vi "Loader.vi"(9 "Loader Name":string, 10 "PID":u32) -> ()   [LabVIEW 2021, in "CIFPluginLoader.lvclass"]
uses:
  CIFPluginLoader.lvclass
  <vilib>/CIF Foundation/CIF Core/CIFUtilities/CIFLogs/Typedef/Message Type.ctl
  gRPC/CIF_PluginLoader_server/RPC Messages/cif_pluginloader_DiscoverResponse.ctl
  gRPC/CIF_PluginLoader_server/RPC Messages/cif_pluginloader_DiscoveredPlugin.ctl
  gRPC/CIF_PluginLoader_server/RPC Messages/cif_common_Version.ctl
  gRPC/CIF_PluginLoader_server/RPC Messages/cif_management_common_PluginMetadata.ctl
  gRPC/CIF_PluginLoader_server/RPC Messages/cif_common_Status.ctl
  CIFPluginLoader.lvclass/CIFPluginLoader.ctl
  gRPC/CIF_PluginLoader_server/RPC Messages/cif_pluginloader_DestroyResponse.ctl
  <vilib>/CIF Foundation/CIF Core/CIFCore/Common/Typedef/Errors.ctl
  gRPC/CIF_PluginLoader_server/RPC Messages/cif_pluginloader_LoadPluginResponse.ctl
  gRPC/CIF_PluginLoader_server/RPC Messages/cif_pluginloader_AbortPluginResponse.ctl
  gRPC/CIF_PluginLoader_server/RPC Messages/cif_pluginloader_PingResponse.ctl
  gRPC/CIF_PluginLoader_server/RPC Messages/cif_management_common_LoaderInfoFull.ctl
  gRPC/CIF_PluginLoader_server/RPC Messages/cif_management_common_LoaderType.ctl
  9a3a4a83-316c-4994-a2ad-738e23b33a77.vi
  903a1d06-a2f6-408e-a72e-d05a96790f6b.vi
  gRPC/CIF_PluginLoader_server/RPC Messages/Get cif_pluginloader_DestroyRequest.vi
  gRPC/CIF_PluginLoader_server/RPC Messages/Set cif_pluginloader_DestroyResponse.vi
  gRPC/CIF_PluginLoader_server/RPC Messages/Get cif_pluginloader_LoadPluginRequest.vi
  gRPC/CIF_PluginLoader_server/RPC Messages/Set cif_pluginloader_LoadPluginResponse.vi
  <vilib>/CIF Foundation/CIF Utilities/Errors/Append Error Location.vi
  gRPC/CIF_PluginLoader_server/RPC Messages/Get cif_pluginloader_AbortPluginRequest.vi
  gRPC/CIF_PluginLoader_server/RPC Messages/Set cif_pluginloader_AbortPluginResponse.vi
  gRPC/CIF_PluginLoader_server/RPC Messages/Get cif_pluginloader_PingRequest.vi
  gRPC/CIF_PluginLoader_server/RPC Messages/Set cif_pluginloader_PingResponse.vi
  gRPC/CIF_PluginLoader_server/RPC Messages/Get cif_pluginloader_DiscoverRequest.vi
  gRPC/CIF_PluginLoader_server/RPC Messages/Set cif_pluginloader_DiscoverResponse.vi
  <vilib>/Utility/High Resolution Relative Seconds.vi
  gRPC/CIF_PluginLoader_server/RPC Messages/Get cif_pluginloader_DestroyRequest.vi/2ed25e12-861d-4677-8ead-ace2906b2041.vi
  gRPC/CIF_PluginLoader_server/RPC Messages/FlatToRichcif_pluginloader_DestroyRequest.vi
  gRPC/CIF_PluginLoader_server/RPC Messages/Set cif_pluginloader_DestroyResponse.vi/dcc74a39-081a-4bdd-860b-8ed792803c96.vi
  gRPC/CIF_PluginLoader_server/RPC Messages/RichToFlatcif_pluginloader_DestroyResponse.vi
  gRPC/CIF_PluginLoader_server/RPC Messages/Get cif_pluginloader_LoadPluginRequest.vi/2ed25e12-861d-4677-8ead-ace2906b2041.vi
  gRPC/CIF_PluginLoader_server/RPC Messages/FlatToRichcif_pluginloader_LoadPluginRequest.vi
  gRPC/CIF_PluginLoader_server/RPC Messages/Set cif_pluginloader_LoadPluginResponse.vi/dcc74a39-081a-4bdd-860b-8ed792803c96.vi
  gRPC/CIF_PluginLoader_server/RPC Messages/RichToFlatcif_pluginloader_LoadPluginResponse.vi
  gRPC/CIF_PluginLoader_server/RPC Messages/Get cif_pluginloader_AbortPluginRequest.vi/2ed25e12-861d-4677-8ead-ace2906b2041.vi
  gRPC/CIF_PluginLoader_server/RPC Messages/FlatToRichcif_pluginloader_AbortPluginRequest.vi
  gRPC/CIF_PluginLoader_server/RPC Messages/Set cif_pluginloader_AbortPluginResponse.vi/dcc74a39-081a-4bdd-860b-8ed792803c96.vi
  gRPC/CIF_PluginLoader_server/RPC Messages/RichToFlatcif_pluginloader_AbortPluginResponse.vi
  gRPC/CIF_PluginLoader_server/RPC Messages/Get cif_pluginloader_PingRequest.vi/2ed25e12-861d-4677-8ead-ace2906b2041.vi
  gRPC/CIF_PluginLoader_server/RPC Messages/FlatToRichcif_pluginloader_PingRequest.vi
  gRPC/CIF_PluginLoader_server/RPC Messages/Set cif_pluginloader_PingResponse.vi/dcc74a39-081a-4bdd-860b-8ed792803c96.vi
  gRPC/CIF_PluginLoader_server/RPC Messages/RichToFlatcif_pluginloader_PingResponse.vi
  gRPC/CIF_PluginLoader_server/RPC Messages/Get cif_pluginloader_DiscoverRequest.vi/2ed25e12-861d-4677-8ead-ace2906b2041.vi
  gRPC/CIF_PluginLoader_server/RPC Messages/FlatToRichcif_pluginloader_DiscoverRequest.vi
  gRPC/CIF_PluginLoader_server/RPC Messages/Set cif_pluginloader_DiscoverResponse.vi/dcc74a39-081a-4bdd-860b-8ed792803c96.vi
  gRPC/CIF_PluginLoader_server/RPC Messages/RichToFlatcif_pluginloader_DiscoverResponse.vi
  <vilib>/gRPC/LabVIEW gRPC Library/Shared/TranslateGrpcError.vi
  gRPC/CIF_PluginLoader_server/RPC Messages/RichToFlatcif_common_Status.vi
  gRPC/CIF_PluginLoader_server/RPC Messages/RichToFlatcif_management_common_LoaderInfoFull.vi
  gRPC/CIF_PluginLoader_server/RPC Messages/RichToFlatcif_pluginloader_DiscoveredPlugin.vi
  gRPC/CIF_PluginLoader_server/RPC Messages/RichToFlatcif_common_Version.vi
  gRPC/CIF_PluginLoader_server/RPC Messages/RichToFlatcif_management_common_PluginMetadata.vi
  <vilib>/gRPC/LabVIEW gRPC Library/Server API/Server/Get Server DLL Path.vi
  <vilib>/Utility/error.llb/Error Cluster From Error Code.vi
  <vilib>/gRPC/LabVIEW gRPC Library/Server API/Message Requests/Complete Call.vi
  <vilib>/gRPC/LabVIEW gRPC Servicer/Servicer/Servicer.lvclass
  <vilib>/CIF Foundation/CIF Core/CIFUtilities/CIFLogs/CIFLogs.lvlib
  <vilib>/Utility/LVLibp/NI_PackedLibraryUtility.lvlib
  gRPC/CIF_PluginLoader_server/RPC Service/PluginLoader/PluginLoader.lvclass
  gRPC/CIF_PluginLoader_server/CIF_PluginLoader_server.lvlib
  gRPC/CIF_Plugin_Loader_Client_Wrapper/CIFPluginLoaderClientWrapper.lvlib
  <vilib>/CIF Foundation/CIF Core/CIFCore/Common/CIFCoreCommon.lvlib
panel:
  out "error out":errorcluster
  in  "stop":bool
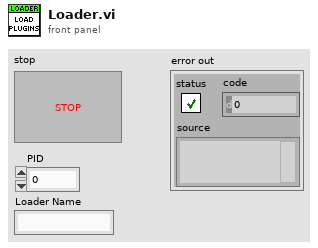
[diagram p1: front panel]
types:
  T1 = typedef "CIFLogs.lvlib/Message Type.ctl" = enum16{"Error", "Information", "Print Terminal", "Configuration"}
  T2 = typedef "CIF_PluginLoader_server.lvlib/cif_pluginloader_DiscoverResponse.ctl" = cluster{"discovered_plugins":T3[], "status":T6}
  T3 = typedef "CIF_PluginLoader_server.lvlib/cif_pluginloader_DiscoveredPlugin.ctl" = cluster{"file_path":string, "file_name":string, "plugin_type":string, "plugin_version":T4, "plugin_metadata":T5, "relative_path":string[]}
  T4 = typedef "CIF_PluginLoader_server.lvlib/cif_common_Version.ctl" = cluster{"major":u32, "minor":u32, "fix":u32, "build":u32}
  T5 = typedef "CIF_PluginLoader_server.lvlib/cif_management_common_PluginMetadata.ctl" = cluster{"description":string, "history":string, "author":string}
  T6 = typedef "CIF_PluginLoader_server.lvlib/cif_common_Status.ctl" = cluster{"code":i32, "message":string}
  T7 = typedef "CIF_PluginLoader_server.lvlib/cif_pluginloader_DestroyResponse.ctl" = cluster{"void":string}
  T8 = typedef "CIFCoreCommon.lvlib/Errors.ctl" = enum16{"Invalid Clock ID", "Long Sleep", "gRPC Server Not Found", "Config Parse", "Timestamp Wrap", "Delayed Execution", "Duplicate Channel", "Missing Channel", "Incorrect Type", "Flatten Error", "Unflatten Data", "Unique Name", "Plugin Not Found", "Plugin Type Not Found", "Plugin Version Not Found", "Manager Not Found", "Numerical Issue", "Time Jump", "Clock ID Match", "Channel Length", "Plugin Connection", "gRPC Server Connection", "PPL Name Match", "Build", "Config Log Parse", "Plugin Load", "UI Subpanel Load", "Python Name", "Invalid Name", "Unable to Change Ch Buffer", "Failed Kill", "Failed SysExec", "Function Not Implemented", "Load Timeout"}
  T9 = typedef "CIF_PluginLoader_server.lvlib/cif_pluginloader_LoadPluginResponse.ctl" = cluster{"status":T6}
  T10 = typedef "CIF_PluginLoader_server.lvlib/cif_pluginloader_AbortPluginResponse.ctl" = cluster{"status":T6}
  T11 = typedef "CIF_PluginLoader_server.lvlib/cif_pluginloader_PingResponse.ctl" = cluster{"loader_info":T12}
  T12 = typedef "CIF_PluginLoader_server.lvlib/cif_management_common_LoaderInfoFull.ctl" = cluster{"loader_type":T13, "loader_name":string, "grpc_port":i32, "pid":u32}
  T13 = typedef "CIF_PluginLoader_server.lvlib/cif_management_common_LoaderType.ctl" = enum32{"LOADERTYPE_UNKNOWN", "LOADERTYPE_LABVIEW"}
  T14 = typedef "grpc-lvsupport-release.lvlib/grpcId.ctl" = u64
  T15 = typedef "CIF_PluginLoader_server.lvlib/cif_pluginloader_LoadPluginRequest.ctl" = cluster{"plugin_name":string, "path":string}
  T16 = typedef "CIFPluginLoader.lvclass/Loaded Plugin Map.ctl" = map{string, refnum<vi>}
  T17 = typedef "CIF_PluginLoader_server.lvlib/cif_pluginloader_AbortPluginRequest.ctl" = cluster{"plugin_name":string}
  T18 = typedef "CIF_Manager_client.lvlib/cif_management_common_LoaderType.ctl" = enum32{"LOADERTYPE_UNKNOWN", "LOADERTYPE_LABVIEW"}
  T19 = typedef "CIF_PluginLoader_server.lvlib/cif_pluginloader_DiscoverRequest.ctl" = cluster{"update_metadata":bool}
  T20 = typedef "CIFPluginManager.lvclass/Discovered Plugin.ctl" = cluster{"Filename":string, "Plugin Type":string, "Qualified name":string, "Version":T21, "Plugin Metadata":T22, "Loader Type":T23, "File Path":string, "Relative Path":string[]}
  T21 = typedef "CIFCoreCommon.lvlib/Version.ctl" = cluster{"Major":i32, "Minor":i32, "Fix":i32, "Build":i32}
  T22 = typedef "CIFPluginManager.lvclass/Plugin Metadata.ctl" = cluster{"Description":string, "History":string, "Author":string}
  T23 = typedef "CIFPluginManager.lvclass/Loader Type.ctl" = enum16{"LabVIEW"}
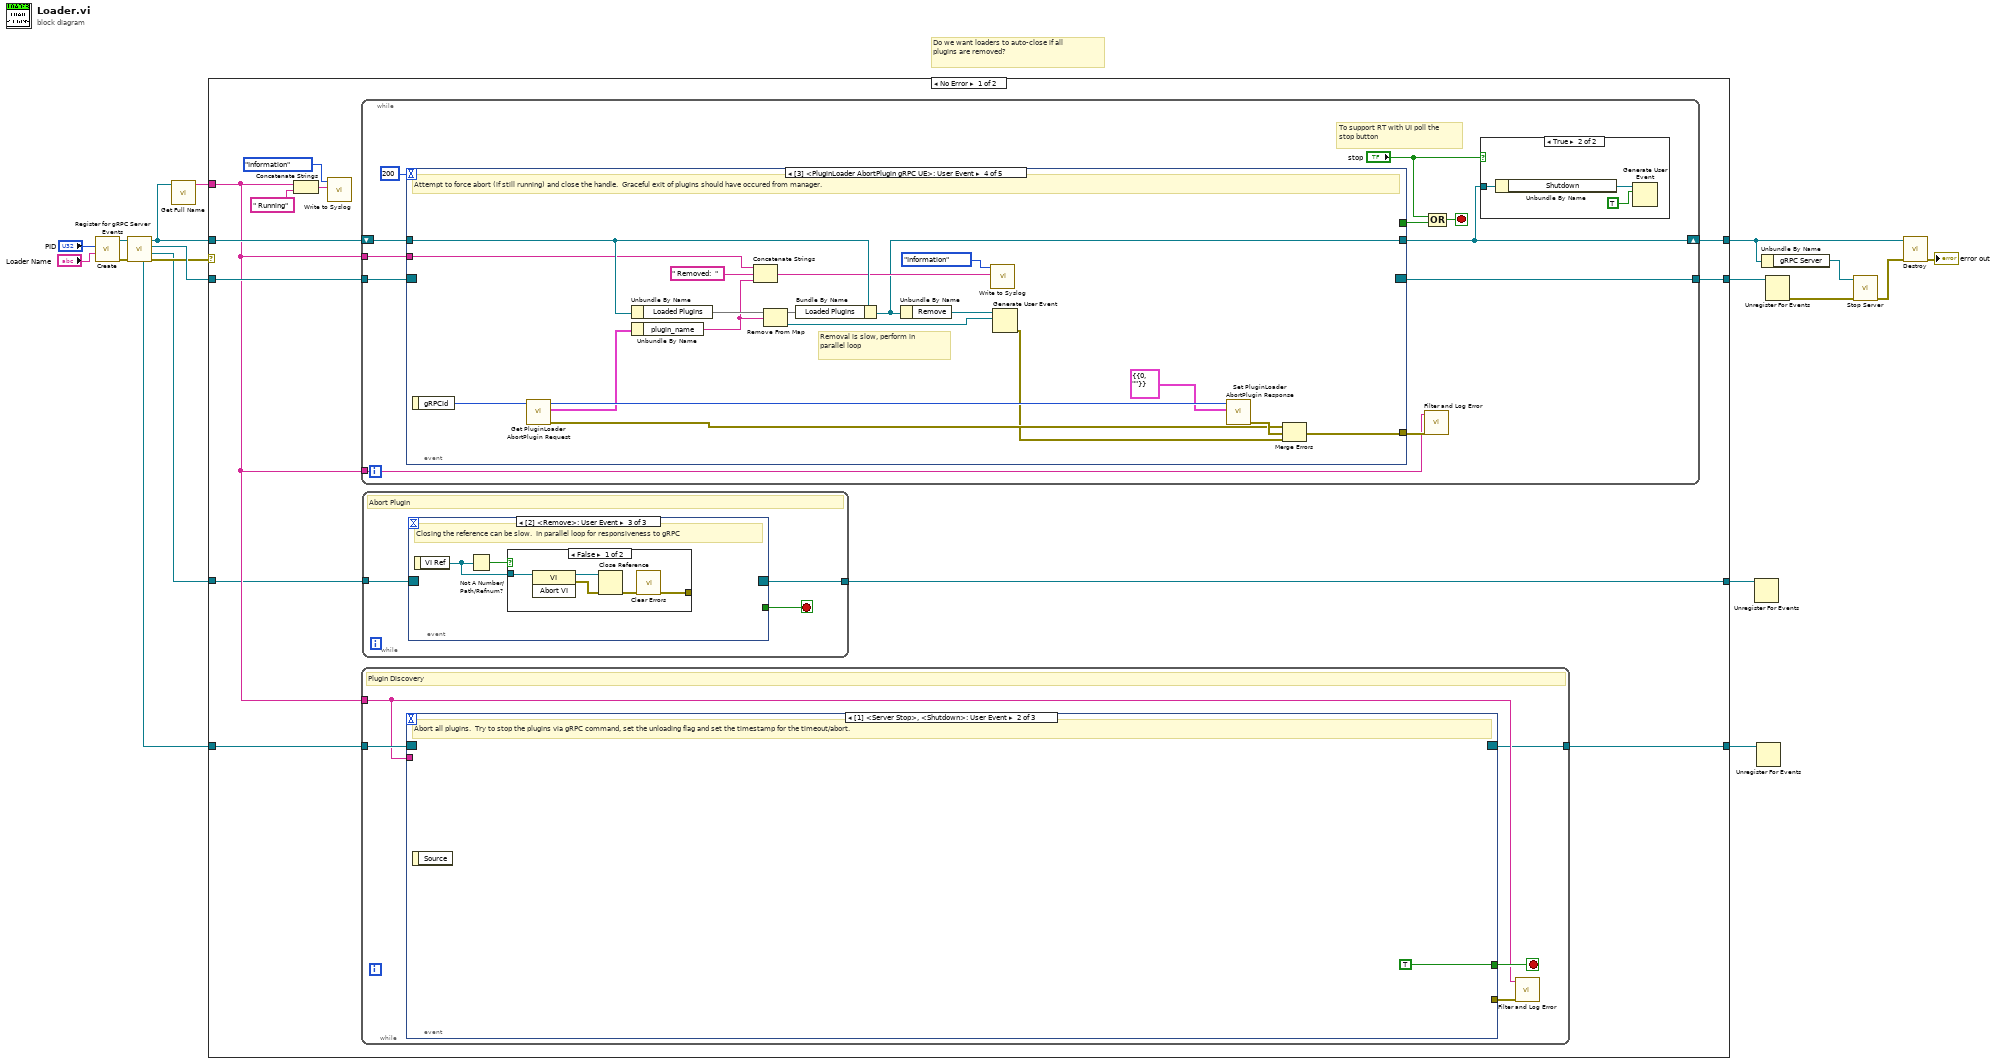
[diagram p0: block diagram]
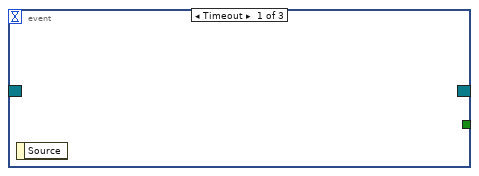
[diagram p2: hidden frame]
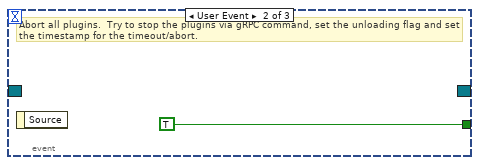
[diagram p3: hidden frame]
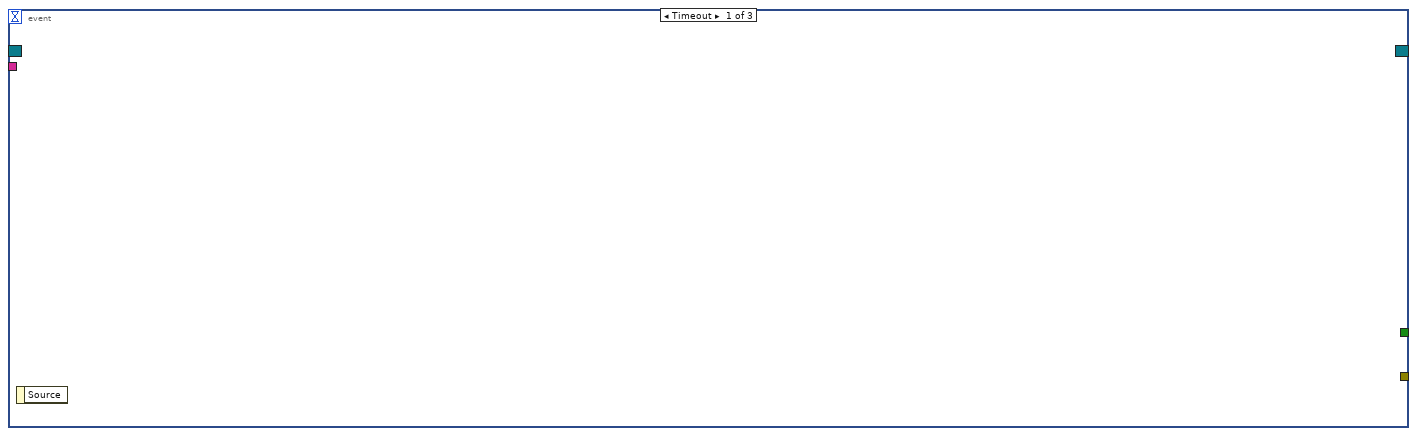
[diagram p5: hidden frame]
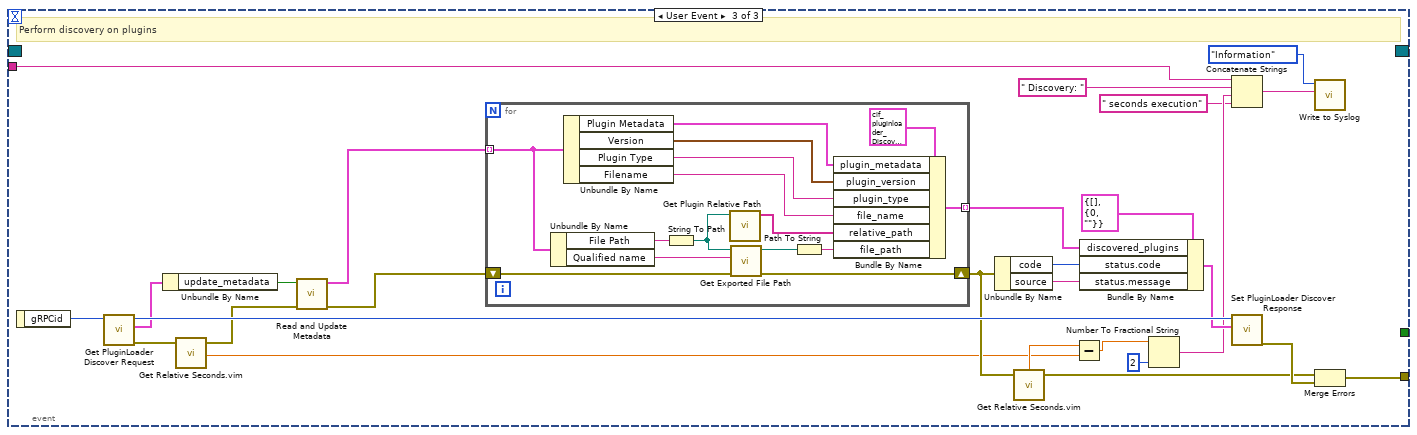
[diagram p6: hidden frame]
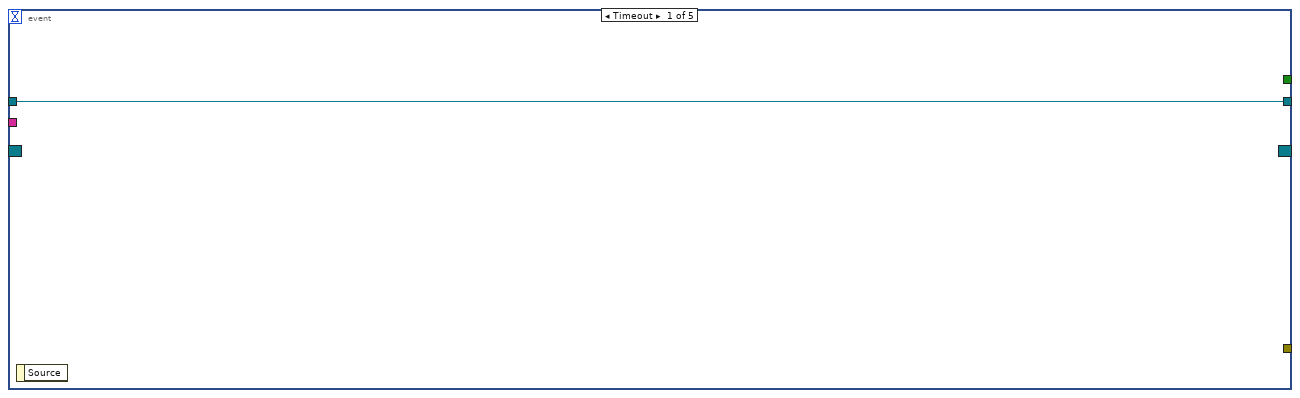
[diagram p8: hidden frame]
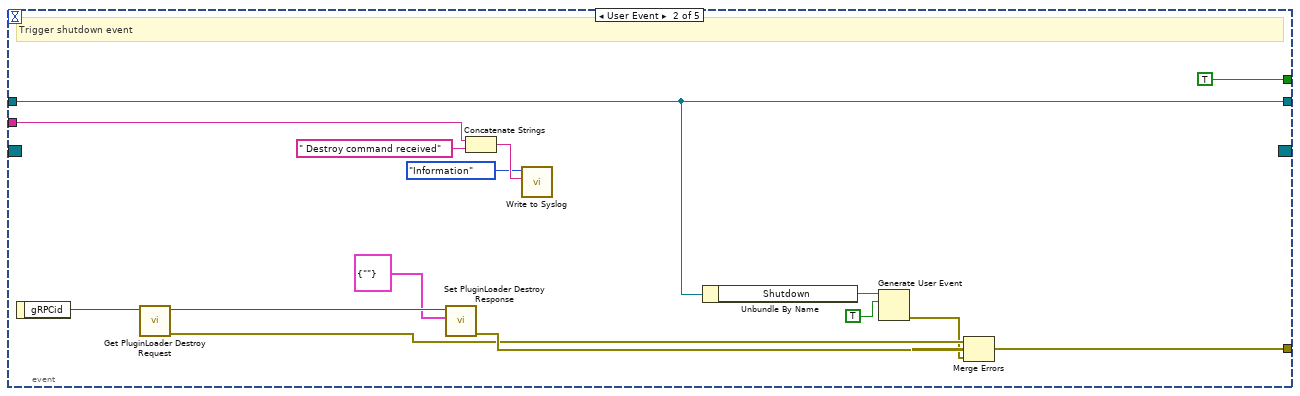
[diagram p9: hidden frame]
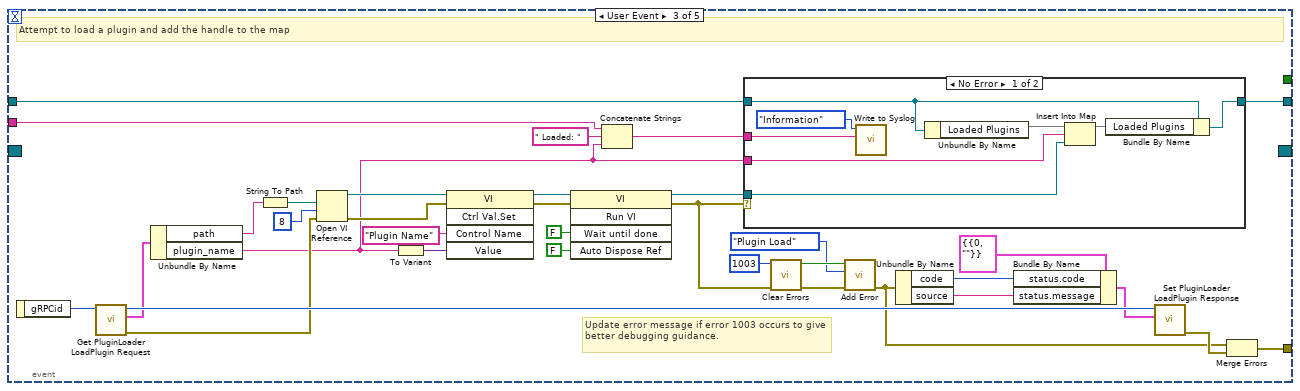
[diagram p10: hidden frame]
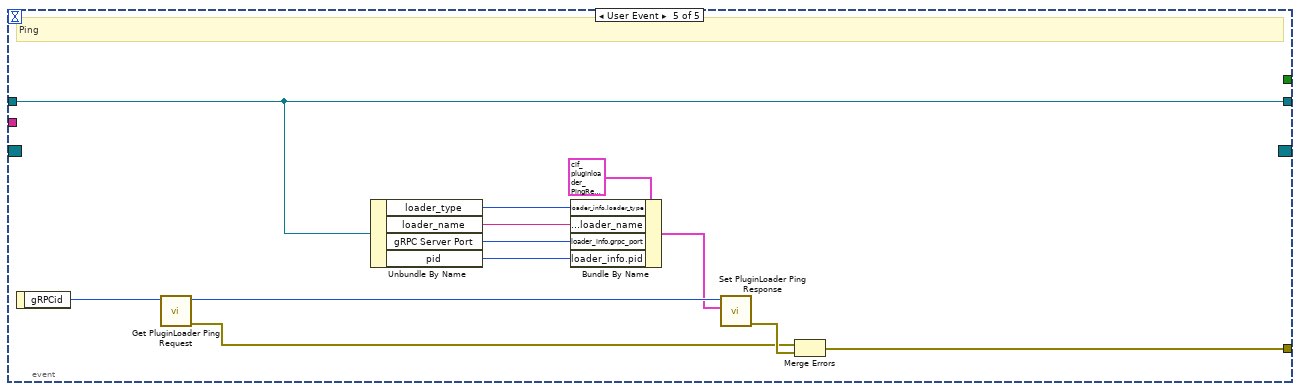
[diagram p12: hidden frame]
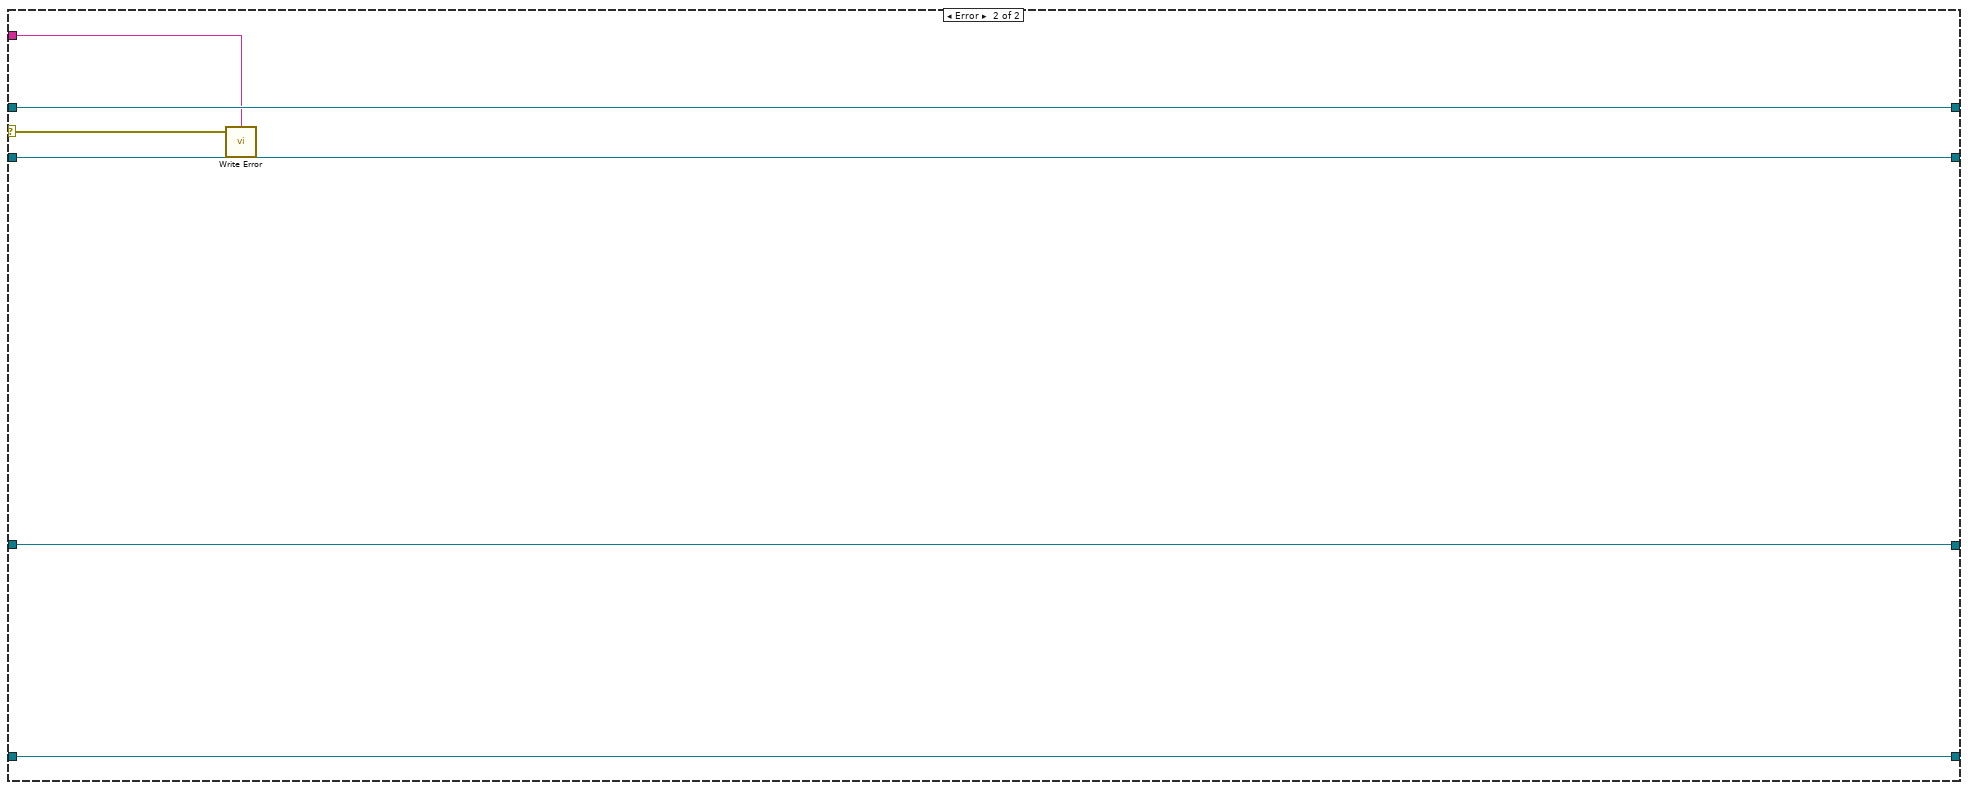
[diagram p13: hidden frame]
diagram:
  # "Do we want loaders to auto-close if all plugins are removed?"
  n1 = call "Create.vi"("Loader Name"="Loader Name", "pid"="PID") -> ("error out"=w13:errorcluster, "Plugin Manager out"=w9:refnum<class "CIFPluginLoader.lvclass">)  [unwired: 8 in]
  n2 = call "Register for gRPC Server Events.vi"("error in (no error)"=w13, "CIFLauncher in"=w9) -> ("error out"=w5:errorcluster, "Abort VI Event Registration Refnum"=w3:refnum<event-registration>, "Main Event Registration Refnum"=w12:refnum<event-registration>, "CIFLauncher out"=w7:refnum<class "CIFPluginLoader.lvclass">, "Discovery Event Registration Refnum"=w4:refnum<event-registration>)  [unwired: 5 in]
  n3 = call "Get Full Name.vi"("CIFPluginLoader in"=w7) -> ("Name"=w6:string)  [unwired: 10 in]
  n4 = case shown="No Error" w5 {
    selector: w5 -> [_ w199]
    tunnel: [w30 w198] -> w8
    tunnel: [w29 w197] -> w14
    tunnel: w12 -> [w28 w197]
    tunnel: w7 -> [w27 w198]
    tunnel: w4 -> [w23 w194]
    tunnel: w6 -> [w22 w196]
    tunnel: w3 -> [w19 w195]
    tunnel: [w21 w194] -> w2
    tunnel: [w20 w195] -> w1
    frame No Error {
      n5 = Concatenate Strings(w22, " Running" ("message")) -> (w26:string)
      n6 = call <vilib>:"Write to Syslog.vi"("message"=w26, "CIF Message Type"=Message_Type."Information") -> ()  [unwired: 9 in, 1 out]
      n7 = while {
        tunnel: w28 -> [w95]
        tunnel: [w99] -> w29
        shift-right: [w98] -> w30
        shift-left: w27 -> [w100]
        tunnel: w22 -> [w94]
        tunnel: w22 -> [w93]
        stop <- w91 stop-if-true
        # "To support RT with UI poll the stop button"
        n8 = event shown="[3] <PluginLoader AbortPlugin gRPC UE>: User Event" {
          selector: w95 -> [_ _ _ _ _]
          dyn-events: [_ _ _ _ _] -> w99
          timeout: 200 -> [_ _ _ _ _]
          tunnel: w100 -> [w104 w106 w136 w175 w186]
          tunnel: [w104 w106 w134 w166 w186] -> w98
          tunnel: [_ w119 w138 w177 w190] -> w97
          tunnel: [_ TRUE _ _ _] -> w92
          tunnel: w93 -> [_ w110 w131 w167 _]
          event Timeout {
            n9 = event-data() -> ()  [unwired: 1 in, 1 out]
          }
          event User Event {
            # "Trigger shutdown event"
            n10 = event-data() -> ("gRPCid"=w117:T14)  [unwired: 1 in]
            n11 = call "Get PluginLoader Destroy Request.vi"("gRPCid"=w117) -> ("error out"=w114:errorcluster, "gRPCid out"=w116:T14)  [unwired: 8 in, 1 out]
            n12 = call "Set PluginLoader Destroy Response.vi"("Message Data"=T7 {"void"=""}, "gRPCid in"=w116) -> ("error out"=w115:errorcluster)  [unwired: 9 in]
            n13 = Concatenate Strings(w110, " Destroy command received" ("message")) -> (w113:string)
            n14 = call <vilib>:"Write to Syslog.vi"("message"=w113, "CIF Message Type"=Message_Type."Information") -> ()  [unwired: 9 in, 1 out]
            n15 = Unbundle By Name(w106) -> ("Shutdown"=w108:refnum<user-event>)
            n16 = Generate User Event(user event=w108, event data cluster=TRUE ("event data")) -> (error out=w105:errorcluster)  [unwired: 2 in, 1 out]
            n17 = Merge Errors(w114, w115, w105) -> (w119:errorcluster)
          }
          event User Event {
            # "Update error message if error 1003 occurs to give better debugging guidance."
            # "Attempt to load a plugin and add the handle to the map"
            n18 = event-data() -> ("gRPCid"=w153:T14)  [unwired: 1 in]
            n19 = call "Get PluginLoader LoadPlugin Request.vi"("gRPCid"=w153) -> ("error out"=w140:errorcluster, "Message Data"=w151:T15, "gRPCid out"=w152:T14)  [unwired: 8 in]
            n20 = Unbundle By Name(w151) -> ("path"=w142:string, "plugin_name"=w128:string)
            n21 = String To Path(string=w142) -> (path=w141:path)
            n22 = Open VI Reference(vi path=w141, options=8, error in (no error)=w140) -> (vi reference=w145:refnum<vi>, error out=w148:errorcluster)  [unwired: 3 in]
            n23 = To Variant(anything=w128) -> (Variant=w143:variant)
            n24 = invoke class="VI" method="Ctrl Val.Set"(reference=w145, error in=w148, "Control Name"="Plugin Name", "Value"=w143) -> (reference out=w147:refnum<vi>, error out=w146:errorcluster)  [unwired: 1 in, 3 out]
            n25 = invoke class="VI" method="Run VI"(reference=w147, error in=w146, "Wait until done"=FALSE ("Wait Until Done"), "Auto Dispose Ref"=FALSE ("Auto Dispose Reference")) -> (reference out=w135:refnum<vi>, error out=w121:errorcluster)  [unwired: 1 in, 3 out]
            n26 = Concatenate Strings(w131, " Loaded: " ("message"), w128) -> (w129:string)
            n27 = case shown="No Error" w121 {
              tunnel: w136 -> [w161 w162]
              tunnel: w128 -> [w159 _]
              tunnel: w135 -> [w158 _]
              tunnel: [w156 w162] -> w134
              tunnel: w129 -> [w154 _]
              frame No Error {
                n28 = call <vilib>:"Write to Syslog.vi"("message"=w154, "CIF Message Type"=Message_Type."Information") -> ()  [unwired: 9 in, 1 out]
                n29 = Unbundle By Name(w161) -> ("Loaded Plugins"=w160:T16)
                n30 = Insert Into Map(map in=w160, key=w159, value=w158) -> (map out=w157:T16)  [unwired: 2 out]
                n31 = Bundle By Name(cluster=w161, "Loaded Plugins"=w157) -> (w156:refnum<class "CIFPluginLoader.lvclass">)
              }
              frame Error {
              }
            }
            n32 = call <vilib>:"Clear Errors.vi"("error in (no error)"=w121, "specific error code to clear (0: all)"=1003) -> ("error out"=w124:errorcluster, "specific error cleared?"=w125:bool)  [unwired: 4 in]
            n33 = call <vilib>:"Add Error.vi"("error in (no error)"=w124, "Error"=Errors."Plugin Load", "Insert Error"=w125) -> ("error out"=w120:errorcluster)  [unwired: 8 in]
            n34 = Unbundle By Name(w120) -> ("code"=w132:i32, "source"=w133:string)
            n35 = Bundle By Name(cluster=T9 {"status"={"code"=0, "message"=""}} ("Message Data"), "status.code"=w132, "status.message"=w133) -> (w127:T9)
            n36 = call "Set PluginLoader LoadPlugin Response.vi"("Message Data"=w127, "gRPCid in"=w152) -> ("error out"=w139:errorcluster)  [unwired: 9 in]
            n37 = Merge Errors(w120, w139) -> (w138:errorcluster)
          }
          event User Event {
            # "Removal is slow, perform in parallel loop"
            # "Attempt to force abort (if still running) and close the handle.  Graceful exit of plugins should have occured from manager."
            n38 = event-data() -> ("gRPCid"=w181:T14)  [unwired: 1 in]
            n39 = call "Get PluginLoader AbortPlugin Request.vi"("gRPCid"=w181) -> ("error out"=w176:errorcluster, "Message Data"=w179:T17, "gRPCid out"=w180:T14)  [unwired: 8 in]
            n40 = Unbundle By Name(w175) -> ("Loaded Plugins"=w173:T16)
            n41 = Unbundle By Name(w179) -> ("plugin_name"=w168:string)
            n42 = Concatenate Strings(w167, " Removed:  " ("message"), w168) -> (w171:string)
            n43 = Remove From Map(10:w168, 11:w173) -> (1:w164:refnum<vi>, 3:w174:T16)  [unwired: 1 out]
            n44 = Bundle By Name(cluster=w175, "Loaded Plugins"=w174) -> (w166:refnum<class "CIFPluginLoader.lvclass">)
            n45 = Unbundle By Name(w166) -> ("Remove"=w165:refnum<user-event>)
            n46 = call <vilib>:"Write to Syslog.vi"("message"=w171, "CIF Message Type"=Message_Type."Information") -> ()  [unwired: 9 in, 1 out]
            n47 = Generate User Event(user event=w165, event data cluster=w164) -> (error out=w163:errorcluster)  [unwired: 2 in, 1 out]
            n48 = call "Set PluginLoader AbortPlugin Response.vi"("Message Data"=T10 {"status"={"code"=0, "message"=""}}, "gRPCid in"=w180) -> ("error out"=w178:errorcluster)  [unwired: 9 in]
            n49 = Merge Errors(w176, w178, w163) -> (w177:errorcluster)
          }
          event User Event {
            # "Ping"
            n50 = event-data() -> ("gRPCid"=w193:T14)  [unwired: 1 in]
            n51 = call "Get PluginLoader Ping Request.vi"("gRPCid"=w193) -> ("error out"=w189:errorcluster, "gRPCid out"=w192:T14)  [unwired: 8 in, 1 out]
            n52 = Unbundle By Name(w186) -> ("loader_type"=w183:T18, "loader_name"=w182:string, "gRPC Server Port"=w188:i32, "pid"=w187:u32)
            n53 = Bundle By Name(cluster=T11 {"loader_info"={"loader_type"=enum."LOADERTYPE_UNKNOWN", "loader_name"="", "grpc_port"=0, "pid"=0}} ("Message Data"), "loader_info.loader_type"=w183, "loader_info.loader_name"=w182, "loader_info.grpc_port"=w188, "loader_info.pid"=w187) -> (w185:T11)
            n54 = call "Set PluginLoader Ping Response.vi"("Message Data"=w185, "gRPCid in"=w192) -> ("error out"=w191:errorcluster)  [unwired: 9 in]
            n55 = Merge Errors(w189, w191) -> (w190:errorcluster)
          }
        }
        n56 = call "Filter and Log Error.vi"("error In"=w97, "Full Name"=w94) -> ()  [unwired: 10 in]
        n57 = Compound Arithmetic op=OR("stop", w92) -> (w91:bool)
        n58 = case shown="True" "stop" {
          tunnel: w98 -> [_ w101]
          frame False {
          }
          frame True {
            n59 = Unbundle By Name(w101) -> ("Shutdown"=w102:refnum<user-event>)
            n60 = Generate User Event(user event=w102, event data cluster=TRUE ("event data")) -> ()  [unwired: 2 in, 2 out]
          }
        }
      }
      n61 = while {
        tunnel: w23 -> [w46]
        tunnel: w22 -> [w43]
        tunnel: [w42] -> w21
        stop <- w45 stop-if-true
        # "Plugin Discovery"
        n62 = event shown="[1] <Server Stop>, <Shutdown>: User Event" {
          selector: w46 -> [_ _ _]
          dyn-events: [_ _ _] -> w42
          timeout: _ -> [_ _ _]
          tunnel: [_ _ w69] -> w44
          tunnel: [_ TRUE _] -> w45
          tunnel: w43 -> [_ _ w52]
          event Timeout {
            n63 = event-data() -> ()  [unwired: 1 in, 1 out]
          }
          event User Event {
            # "Abort all plugins.  Try to stop the plugins via gRPC command, set the unloading flag and set the timestamp for the timeout/abort."
            n64 = event-data() -> ()  [unwired: 1 in, 1 out]
          }
          event User Event {
            # "Perform discovery on plugins"
            n65 = event-data() -> ("gRPCid"=w74:T14)  [unwired: 1 in]
            n66 = call "Get PluginLoader Discover Request.vi"("gRPCid"=w74) -> ("error out"=w62:errorcluster, "Message Data"=w72:T19, "gRPCid out"=w73:T14)  [unwired: 8 in]
            n67 = Unbundle By Name(w72) -> ("update_metadata"=w71:bool)
            n68 = call "Get Relative Seconds.vim"("Anything in"=w62) -> ("Relative Seconds"=w57:dbl, "Anything out"=w61:errorcluster)  [unwired: 2 in]
            n69 = call "Read and Update Metadata.vi"("error in (no error)"=w61, "Update Metadata"=w71) -> ("error out"=w67:errorcluster, "Plugin Info"=w68:T20[])  [unwired: 8 in]
            n70 = for {
              tunnel: w68 -> [w87] mode=indexing
              shift-right: [w88] -> w60
              shift-left: w67 -> [w89]
              tunnel: [w80] -> w65 mode=indexing
              n71 = Unbundle By Name(w87) -> ("File Path"=w77:string, "Qualified name"=w79:string)
              n72 = Unbundle By Name(w87) -> ("Plugin Metadata"=w81:T22, "Version"=w82:T21, "Plugin Type"=w83:string, "Filename"=w84:string)
              n73 = String To Path(string=w77) -> (path=w76:path)
              n74 = call "Get Plugin Relative Path.vi"("File Path"=w76) -> ("Relative Path"=w75:string[])  [unwired: 10 in]
              n75 = call <vilib>:"Get Exported File Path.vi"("error in (no error)"=w89, "qualified name"=w79, "packed library path"=w76) -> ("error out"=w88:errorcluster, "path"=w86:path)  [unwired: 7 in]
              n76 = Path To String(path=w86) -> (string=w85:string)
              n77 = Bundle By Name(cluster=T3 {"file_path"="", "file_name"="", "plugin_type"="", "plugin_version"={"major"=0, "minor"=0, "fix"=0, "build"=0}, "plugin_metadata"={"description"="", "history"="", "author"=""}, "relative_path"=[]} ("cif_pluginloader_DiscoveredPlugin"), "plugin_metadata"=w81, "plugin_version"=w82, "plugin_type"=w83, "file_name"=w84, "relative_path"=w75, "file_path"=w85) -> (w80:T3)
            }
            n78 = Unbundle By Name(w60) -> ("code"=w66:i32, "source"=w64:string)
            n79 = call "Get Relative Seconds.vim"("Anything in"=w60) -> ("Relative Seconds"=w58:dbl, "Anything out"=w59:errorcluster)  [unwired: 2 in]
            n80 = Subtract(x=w58, y=w57) -> (x-y=w56:dbl)
            n81 = Bundle By Name(cluster=T2 {"discovered_plugins"=[], "status"={"code"=0, "message"=""}} ("Message Data"), "discovered_plugins"=w65, "status.code"=w66, "status.message"=w64) -> (w63:T2)
            n82 = Number To Fractional String(number=w56, precision (6)=i16 2) -> (F-format string=w51:string)  [unwired: 2 in]
            n83 = Concatenate Strings(w52, " Discovery: " ("message"), w51, " seconds execution" ("message")) -> (w55:string)
            n84 = call "Set PluginLoader Discover Response.vi"("Message Data"=w63, "gRPCid in"=w73) -> ("error out"=w70:errorcluster)  [unwired: 9 in]
            n85 = call <vilib>:"Write to Syslog.vi"("message"=w55, "CIF Message Type"=Message_Type."Information") -> ()  [unwired: 9 in, 1 out]
            n86 = Merge Errors(w59, w70) -> (w69:errorcluster)
          }
        }
        n87 = call "Filter and Log Error.vi"("error In"=w44, "Full Name"=w43) -> ()  [unwired: 10 in]
      }
      n88 = while {
        tunnel: [w33] -> w20
        tunnel: w19 -> [w32]
        stop <- w31 stop-if-true
        # "Abort Plugin"
        n89 = event shown="[2] <Remove>: User Event" {
          selector: w32 -> [_ _ _]
          dyn-events: [_ _ _] -> w33
          timeout: _ -> [_ _ _]
          tunnel: [_ TRUE _] -> w31
          event Timeout {
            n90 = event-data() -> ()  [unwired: 1 in, 1 out]
          }
          event User Event {
            # "Abort all plugins.  Try to stop the plugins via gRPC command, set the unloading flag and set the timestamp for the timeout/abort."
            n91 = event-data() -> ()  [unwired: 1 in, 1 out]
          }
          event User Event {
            # "Closing the reference can be slow.  In parallel loop for responsiveness to gRPC"
            n92 = event-data() -> ("VI Ref"=w35:refnum<vi>)  [unwired: 1 in]
            n93 = Not A Number/Path/Refnum?(number/path/refnum=w35) -> (NaN/Path/Refnum?=w36:bool)
            n94 = case shown="False" w36 {
              tunnel: w35 -> [w39 _]
              tunnel: [w40 _] -> _
              frame False {
                n95 = invoke class="VI" method="Abort VI"(reference=w39) -> (reference out=w38:refnum<vi>, error out=w37:errorcluster)  [unwired: 2 in, 1 out]
                n96 = Close Reference(reference=w38, error in (no error)=w37) -> (error out=w41:errorcluster)
                n97 = call <vilib>:"Clear Errors.vi"("error in (no error)"=w41) -> ("error out"=w40:errorcluster)  [unwired: 5 in, 1 out]
              }
              frame True {
              }
            }
          }
        }
      }
    }
    frame Error {
      n98 = call <vilib>:"Write Error.vi"("error in (no error)"=w199, "Plugin Name"=w196) -> ()  [unwired: 2 in, 1 out]
    }
  }
  n99 = Unregister For Events(event registration refnum=w1) -> ()  [unwired: 1 in, 1 out]
  n100 = Unregister For Events(event registration refnum=w2) -> ()  [unwired: 1 in, 1 out]
  n101 = Unbundle By Name(w8) -> ("gRPC Server"=w17:refnum<class "Servicer.lvclass">)
  n102 = Unregister For Events(event registration refnum=w14) -> (error out=w18:errorcluster)  [unwired: 1 in]
  n103 = call <vilib>:"Stop Server.vi"("error in"=w18, "gRPC server in"=w17) -> ("error out"=w16:errorcluster)  [unwired: 9 in]
  n104 = call "Destroy.vi"("error in (no error)"=w16, "Plugin Manager in"=w8) -> ("error out"=→"error out":errorcluster)  [unwired: 8 in, 1 out]
